vi "Monitor Queue Status to DBLs.vi"(3 "MonQueueStatus":T1 {"QueueStatus" items=["FDX_MON_STAT_EMPTY", "FDX_MON_STAT_ FILLED", "FDX_MON_STAT_ FULL", "FDX_MON_STAT_ OVERFLOW", "FDX_MON_STAT_ ERROR"]}) -> (1 "MonQueueStatusDBLs":dbl[](array[numeric]))   [LabVIEW 2020, in "AIM ARINC 664 Engine.lvlib" / "Implementation.lvlib" / "Monitor Execution Unit.lvclass"]
uses:
  Monitor Execution Unit.lvclass
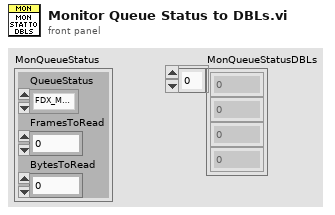
[diagram p1: front panel]
types:
  T1 = cluster{"QueueStatus":u32, "FramesToRead":u32, "BytesToRead":u32}
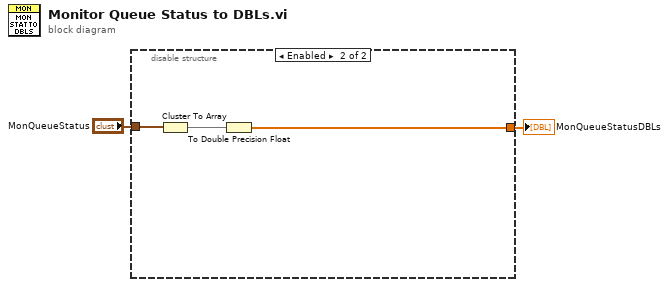
[diagram p0: block diagram]
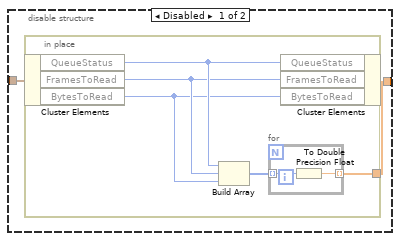
[diagram p2: hidden frame]
diagram:
  n1 = disable-structure shown="Enabled" {
    disable-tunnel: [w4 w12] -> w2
    disable-tunnel: "MonQueueStatus" -> [w3 w14]
    frame Disabled {
      n2 = in-place {
        in-place-border: [w5] -> w4
        n3 = in-place-cluster #1(w3) -> ("QueueStatus"=w9:u32, "FramesToRead"=w8:u32, "BytesToRead"=w7:u32)
        n4 = Build Array(w9, w8, w7) -> (w6:u32[])
        n5 = for {
          tunnel: w6 -> [w11] mode=indexing
          tunnel: [w10] -> w5 mode=indexing
          n6 = To Double Precision Float(number=w11) -> (double precision float=w10:dbl)
        }
        n7 = in-place-cluster #1("QueueStatus"=w9, "FramesToRead"=w8, "BytesToRead"=w7) -> ()  [unwired: 1 out]
      }
    }
    frame Enabled {
      n8 = Cluster To Array(cluster=w14) -> (array=w13:u32[])
      n9 = To Double Precision Float(number=w13) -> (double precision float=w12:dbl[])
    }
  }
  "MonQueueStatusDBLs" <- w2
